vi "NI 5772 (AC) - TIS Mode Enabled (Host).vi"() -> ()   [LabVIEW 2020]
doc: "Example Description:\nThis example demonstrates how to enable Time Interleaved Sampling with the NI 5772 adapter module to achieve a sampling rate of 1.6GS/s. This example continuously acquires records of analog input data from the NI 5772 adapter module. It allows you to select an AI channel, trigger type, and record size. This VI must be compiled before it is run. \n\nVI Configuration:\nThis example uses the NI PXI-7952R as the FPGA target by default. If you are using another FPGA target, complete the following steps to configure the host VI to use a VI configured for your FPGA target:\n1. On the block diagram, right-click the Open FPGA VI Reference (NI PXI-7952R) function and select Configure Open FPGA VI Reference.\n2. Browse for a new target by clicking the Browse Project button in the Open VI section.\n3. Select the VI under the target that matches your device. Click OK to select this VI.\n4. Click OK to exit the dialog box and to apply the new selection to the FPGA VI.\n5. Save the VI.\n\nRunning the VI:\n1. Select a RIO Resource that corresponds to the FPGA device configured above.\n2. Clock Configuration: Select the desired clock source for the adapter module.\nAnalog Input: Configure the AI Channel, Record Size, and Trigger Type controls. If you are using the analog trigger type, configure the Trigger Level (V) control.\n3. Click the run arrow to run the VI.\n4. If the Trigger Type is set to Software, click the Software Trigger button to acquire a single record of data. If the Trigger Type is set to Data Edge, a record of data is acquired each time the input signal rises above the trigger level.\n\nThe Record Size, Trigger Type, and Trigger Level (V) controls can all be configured while the VI is running. \n\nNote: The AI Channel control must be configured before the VI is run.\n\nExecution Steps:s\n1. Open a session to the FPGA VI and run the VI.\n2. Wait for the adapter module to load its default configuration.\n3. Configure the NI 5772 for Time Interleaved Sampling (TIS)\n4. The Trigger type and record size for a single record acquisition are configured.\n5. Based on the trigger type, either wait for the software trigger Boolean to assert or configure the desired trigger level and arm the trigger.\n6. After the trigger is armed, a single record of data is acquired and read.\n7. Stop the VI when the stop button is pressed or when an error has occurred. \n8. Close the FPGA VI reference and display any errors."
uses:
  <vilib>/userdefined/High Color/nirio_resource_hc.ctl
  Digi/Controls/TIS Mode.ctl
  <vilib>/FPGAPlugInAG/PXIe-7962R/niLvFpga_Open_PXIe-7962R.vi
  <vilib>/rvi/interface/common/dynamic/niFpgaDynamicAddResources.vi
  <vilib>/Utility/error.llb/Error Cluster From Error Code.vi
  <vilib>/rvi/errors/niLvFpgaAdjustHostInterfaceError.vi
  <instrlib>/_niInstr/Basic Elements/v1/FPGA/Private/Count Up U8.vi
  <vilib>/FPGAPlugInAG/Dynamic/niLvFpga_Close_Dynamic.vi
  <vilib>/rvi/interface/nirviOpenFPGA/nirviOpenFPGA.xnode
  FPGA Bitfiles/acoustoxv3_FPGATarget_OriginalDigitize_EOlkFE5eWpM.lvbitx
  Digi/OriginalDigitizerLive.vi
  <vilib>/rvi/interface/nirviReadWriteControl/nirviReadWriteControl.xnode
  <vilib>/rvi/interface/nirviMethod/nirviMethod.xnode
  <vilib>/rvi/interface/nirviCloseFPGA/nirviCloseFPGA.xnode
  NiFpgaLv.dll
  <vilib>/rvi/interface/Simulation/niFpgaSimulationCallBeginRW.vi
  <vilib>/FPGAPlugInAG/Dynamic/niLvFpga_ReadFifo_Dynamic.vi
  <vilib>/rvi/errors/niLvFpgaMergeErrorWithErrorCode.vi
  <instrlib>/_niInstr/Basic Elements/v1/FPGA/niInstr Basic Elements v1 FPGA.lvlib
panel:
  in  "vi/nGenTrig":bool
  out "Acquire State":T1(ring)
  in  "WaitForWave Completion [cycles]":u16
  out "Avg State":T2(ring)
  out "count out":u8
  in  "AvgCount_powerOf2":i16
  out "Analog Input 2":i16[](graph) caption="Acquired Waveform"
  in  "Delay Cycles":u16
  out "Mean":dynamicdata(graph)
  in  "DS":u8
  out "Elements Remaining":u32
  out "Requested":u16
  in  "TIS Mode":T3=3 items=["TIS Mode (CH0 Only)"=1, "TIS Mode (CH1 Only)"=2, "Dual TIS Mode (CH0 and CH1)"=3]
  out "TIS Configured?":bool
  out "Analog Input":cluster{"Start Time":dbl, dbl, ext[]}(graph) caption="Acquired Waveform"
  out "error out":errorcluster
  in  "stop":bool
  in  "Trigger Level (V)":dbl
  in  "Software Trigger":bool
  in  "Record Size":u16=1024
  in  "Trigger Type":enum8{"Software", "Data Edge"}(ring)
  in  "RIO Resource":T4="PXI1Slot2"
  out "Configured?":bool
  # "Resource Configuration"
  # "AI Configuration"
  # "Interleaved Configuration"
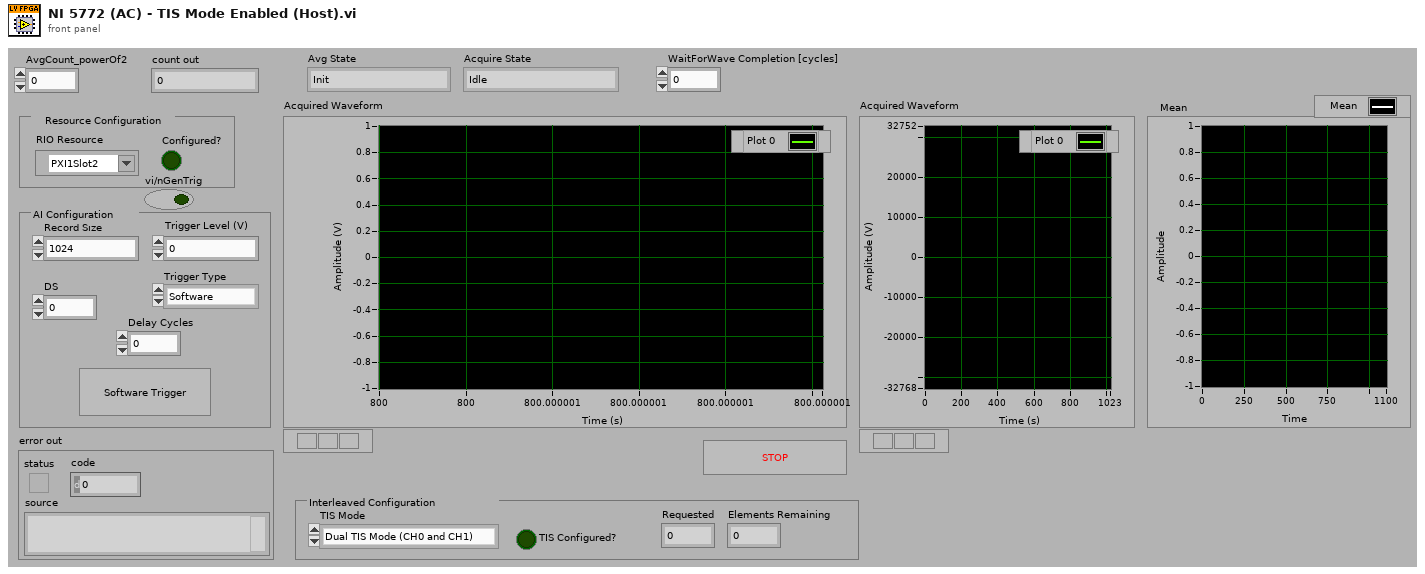
[diagram p1: front panel]
types:
  T1 = enum8{"Idle", "Wait for Trigger", "AlignWave", "Hold Aquire", "Acquire", "WaitForWaveCompletion", "CheckAvg"}
  T2 = enum16{"Init", "Clear Accumulator", "Build Accumulator", "GetData", "SetData", "AverageCountCheck", "SendtoHost"}
  T3 = typedef "TIS Mode.ctl" = u16
  T4 = typedef "nirio_resource_hc.ctl" = tag
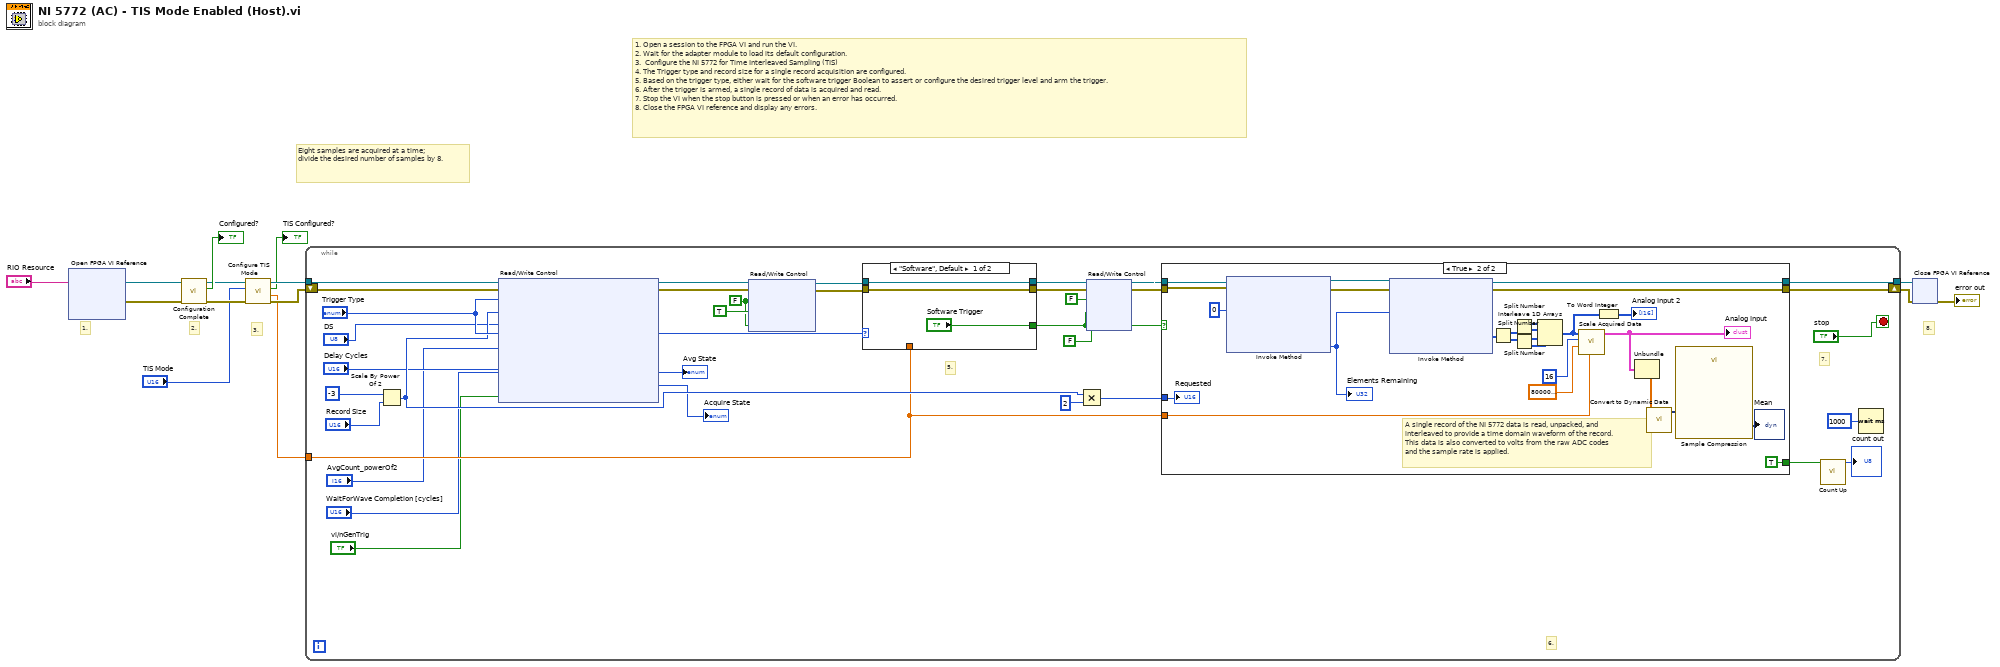
[diagram p0: block diagram]
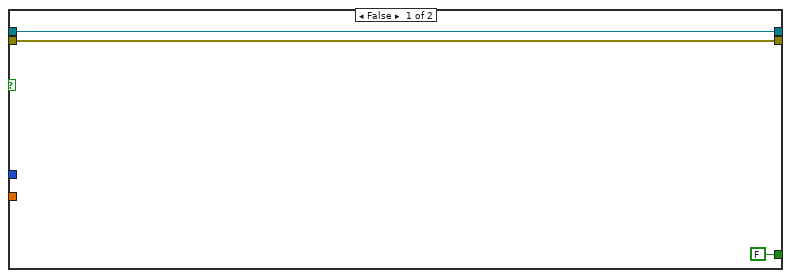
[diagram p2: hidden frame]
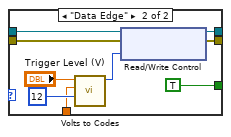
[diagram p3: hidden frame]
diagram:
  # "Eight samples are acquired at a time; divide the desired number of samples by 8."
  # "8."
  # "3."
  # "2."
  # "1."
  # "1. Open a session to the FPGA VI and run the VI.\n2. Wait for the adapter module to load its default configuration.\n3.  Configure the NI 5772 for Time Interleaved Sampling (TIS)\n4. The Trigger type and record size for a single record acquisition are configured.\n5. Based on the trigger type, either wait for the software trigger Boolean to assert or configure the desired trigger level and arm the trigger.\n6. After the trigger is armed, a single record of data is acquired and read.\n7. Stop the VI when the stop button is pressed or when an error has occurred.  \n8. Close the FPGA VI reference and display any errors."
  n1 = xnode "Open FPGA VI Reference"("resource name"="RIO Resource") -> ("FPGA VI Reference Out"=w1:refnum<k20>, "error out"=w10:errorcluster)  [unwired: 1 in]
  n2 = call "Configuration Complete.vi"("error in"=w10, "FPGA VI Reference In"=w1) -> ("error out"=w9:errorcluster, "Configured?"=→"Configured?":bool, "FPGA VI Reference Out"=w7:refnum<k20>)  [unwired: 7 out]
  n3 = call "Configure TIS Mode.vi"("error in"=w9, "TIS Mode"="TIS Mode", "FPGA VI Reference In"=w7) -> ("error out"=w8:errorcluster, "range (Vpp)"=w2:dbl, "TIS Configured?"=→"TIS Configured?":bool, "FPGA VI Reference Out"=w6:refnum<k20>)  [unwired: 5 in]
  n4 = while {
    tunnel: [w48] -> w13
    tunnel: w6 -> [w42]
    shift-right: [w43] -> w11
    shift-left: w8 -> [w41]
    tunnel: w2 -> [w36]
    stop <- "stop" stop-if-true
    w16 = FALSE ("Arm Trigger")
    # "7."
    # "6."
    # "5."
    n5 = Scale By Power Of 2(n=-3, x="Record Size") -> (x*2^n=w37:u16)
    n6 = xnode "Read/Write Control"("FPGA VI Reference In"=w42, "error in"=w41, "Trigger Type"="Trigger Type", "Samples Per Trigger"=w37, "DS"="DS", "Delay Cycles"="Delay Cycles", "AvgCount_powerOf2"="AvgCount_powerOf2", "WaitForWave Completion [cycles]"="WaitForWave Completion [cycles]", "vi/nGenTrig"="vi/nGenTrig") -> ("FPGA VI Reference Out"=w21:refnum<k20>, "error out"=w20:errorcluster, "Avg State"=→"Avg State":T2, "Acquire State"=→"Acquire State":T1)
    n7 = xnode "Read/Write Control"("FPGA VI Reference In"=w21, "error in"=w20, "Arm Trigger"=w16, "Arm Trigger"=TRUE, "Arm Trigger"=w16) -> ("FPGA VI Reference Out"=w19:refnum<k20>, "error out"=w18:errorcluster)
    n8 = case shown="\"Software\", Default" "Trigger Type" {
      tunnel: w19 -> [w81 w90]
      tunnel: w18 -> [w80 w89]
      tunnel: [w81 w88] -> w47
      tunnel: [w80 w87] -> w46
      tunnel: ["Software Trigger" TRUE ("Acquire")] -> w32
      tunnel: w36 -> [_ w82]
      frame "Software", Default {
      }
      frame "Data Edge" {
        n9 = call "Volts to Codes.vi"("Number of Bits"=i16 12, "range (Vpp)"=w82, "Data In"="Trigger Level (V)") -> ("Data Out"=w83:i16)  [unwired: 8 out]
        n10 = xnode "Read/Write Control"("FPGA VI Reference In"=w90, "error in"=w89, "Trigger Level"=w83) -> ("FPGA VI Reference Out"=w88:refnum<k20>, "error out"=w87:errorcluster)
      }
    }
    n11 = Multiply(x=w37, y=u16 2) -> (x*y=w35:u16)
    n12 = xnode "Read/Write Control"("FPGA VI Reference In"=w47, "error in"=w46, "Trigger"=FALSE, "Trigger"=w32, "Trigger"=FALSE) -> ("FPGA VI Reference Out"=w45:refnum<k20>, "error out"=w44:errorcluster)
    n13 = case shown="True" w32 {
      tunnel: w45 -> [w51 w62]
      tunnel: w44 -> [w52 w63]
      tunnel: [w52 w78] -> w43
      tunnel: [w51 w77] -> w48
      tunnel: w35 -> [_ w66]
      tunnel: w36 -> [_ w74]
      tunnel: [FALSE ("increment") TRUE ("increment")] -> w26
      frame False {
      }
      frame True {
        # "A single record of the NI 5772 data is read, unpacked, and interleaved to provide a time domain waveform of the record. This data is also converted to volts from the raw ADC codes and the sample rate is applied."
        n14 = xnode "Invoke Method"("FPGA VI Reference In"=w62, "error in"=w63, "Number of Elements"=u32 0) -> ("FPGA VI Reference Out"=w65:refnum<k20>, "error out"=w64:errorcluster, "Elements Remaining"=w61:u32)  [unwired: 1 in, 1 out]
        "Elements Remaining" <- w61
        n15 = xnode "Invoke Method"("FPGA VI Reference In"=w65, "error in"=w64, "Number of Elements"=w61) -> ("FPGA VI Reference Out"=w77:refnum<k20>, "error out"=w78:errorcluster, "Data"=w73:u64[])  [unwired: 1 in, 1 out]
        n16 = Split Number(x=w73) -> (hi(x)=w72:u32[], lo(x)=w71:u32[])
        n17 = Split Number(x=w72) -> (hi(x)=w70:u16[], lo(x)=w67:u16[])
        n18 = Split Number(x=w71) -> (hi(x)=w68:u16[], lo(x)=w69:u16[])
        n19 = Interleave 1D Arrays(w70, w67, w68, w69) -> (w55:u16[])
        n20 = call "Scale Acquired Data.vi"("range (V)"=w74, "Sample Rate"=800000000.0, "Number of Bits"=i16 16, "Data In"=w55) -> ("output waveform"=w59:cluster{"Start Time":dbl, dbl, ext[]})  [unwired: 1 in, 6 out]
        "Analog Input" <- w59
        n21 = To Word Integer(number=w55) -> (16bit integer=→"Analog Input 2":i16[])
        n22 = Unbundle(w59) -> (w58:ext[])  [unwired: 2 out]
        n23 = call "Convert to Dynamic Data"("Array"=w58) -> ("Dynamic Data Type"=w57:dynamicdata)  [unwired: 3 in]
        n24 = call "Sample Compression"("Signals"=w57) -> ("Mean"=→"Mean":dynamicdata)  [unwired: 8 in, 2 out]
        "Requested" <- w66
      }
    }
    n25 = call-poly <instrlib>:"Count Up.vi"("increment"=w26) -> ("count out"=→"count out":u8)  [unwired: 14 in]
    n26 = Wait (ms)(milliseconds to wait=u32 1000) -> ()  [unwired: 1 out]
  }
  n27 = xnode "Close FPGA VI Reference"("FPGA VI Reference In"=w13, "error in"=w11) -> ("error out"=→"error out":errorcluster)
